vi "VMI_queue_clean_up_arrays.vi"(2 "error in (no error)":errorcluster, 3 "Queue Array":T1[](array[typedef])) -> (0 "error out":errorcluster)   [LabVIEW 2020]
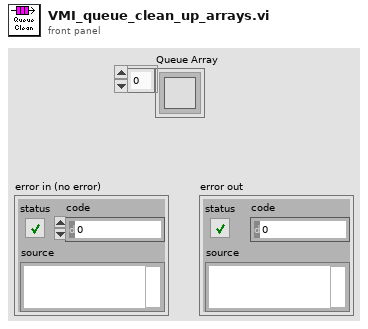
[diagram p1: front panel]
types:
  T1 = typedef "Queue RefNum" = refnum<k1>
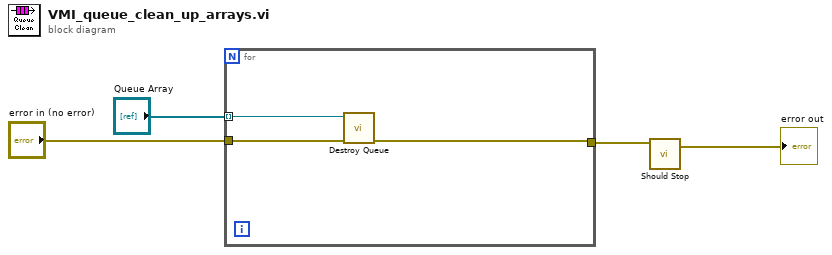
[diagram p0: block diagram]
diagram:
  n1 = for {
    tunnel: "Queue Array" -> [w7] mode=indexing
    tunnel: "error in (no error)" -> [w6]
    tunnel: [w5] -> w2
    n2 = call <vilib>:"Destroy Queue.vi"("error in (no error)"=w6, "queue"=w7) -> ("error out"=w5:errorcluster)  [unwired: 3 in, 2 out]
  }
  n3 = call "Should Stop.vi"("error in 1"=w2) -> ("error out"=→"error out":errorcluster)  [unwired: 4 in, 1 out]
